vi "Toggle Sub BG.vi"(8 "error in (no error)":errorcluster, 11 "IMAQ Display in":refnum<class "HIJ IMAQdx Display.lvclass">) -> (0 "error out":errorcluster, 3 "IMAQ Display out":refnum<class "HIJ IMAQdx Display.lvclass">)   [LabVIEW 2014, in "HIJ IMAQdx Display.lvlib" / "HIJ IMAQdx Display.lvclass"]
uses:
  HIJ IMAQdx Display.lvclass
  HIJ IMAQdx Display.lvclass/HIJ IMAQdx Display.ctl
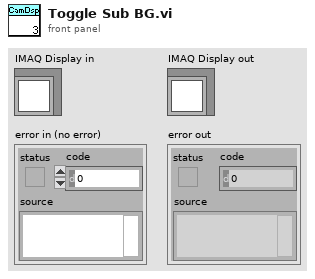
[diagram p1: front panel]
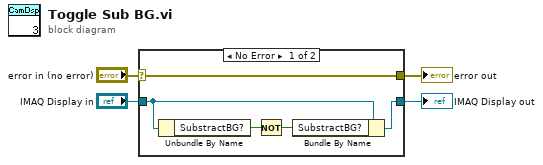
[diagram p0: block diagram]
diagram:
  n1 = case shown="No Error" "error in (no error)" {
    selector: "error in (no error)" -> [w9 w11]
    tunnel: [w9 w11] -> w3
    tunnel: [w5 w10] -> w1
    tunnel: "IMAQ Display in" -> [w6 w10]
    frame No Error {
      n2 = Unbundle By Name(w6) -> ("SubstractBG?"=w7:bool)
      n3 = Not(x=w7) -> (.not. x?=w8:bool)
      n4 = Bundle By Name(cluster=w6, "SubstractBG?"=w8) -> (w5:refnum<class "HIJ IMAQdx Display.lvclass">)
    }
    frame Error {
    }
  }
  "error out" <- w3
  "IMAQ Display out" <- w1
